vi "Global Zero or Not Ctrl.vi"() -> ()   [LabVIEW 2020]
panel:
  in  "State":string="Print"
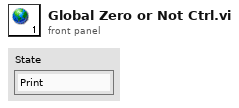
[diagram p1: front panel]
diagram:
